vi "rus fit - write RPR line.vi"(9 "folder path":path, 11 "lorentzian":T1={"Amplitude"=0.0035518868945241954, "omega(0)"=2372.1004391165757, "Gamma"=0.8336723020896565, "phase"=3.2843535262399524, "Q"=2845.3631398941097, "Norm  Ampl"=0.37874134839899876, "z (inf)"=0.04739549353095661-0.43244178436899827i, "4corners"={"z (-pi/2)"=-0.4669245429896878-0.04739549353095661i, "z(inf)"=0.04739549353095661-0.43244178436899827i, "z (pi/2)"=0.43244178436899827+0.08187825215164611i, "z center"=-0.01724137931034475+0.01724137931034475i, "z(0)"=-0.08187825215164611+0.4669245429896878i, "radius"=0.45430482390941584}} {"z (inf)" format="%#9_9f"; "Q" format="%#9_9f"; "phase" format="%#9_9f"; "Gamma" format="%#9_9f"; "omega(0)" format="%#9_9f"}) -> ()   [LabVIEW 2015]
uses:
  lorentzian.ctl
  circle corners.ctl
  <vilib>/Utility/file.llb/Write To Spreadsheet File (string).vi
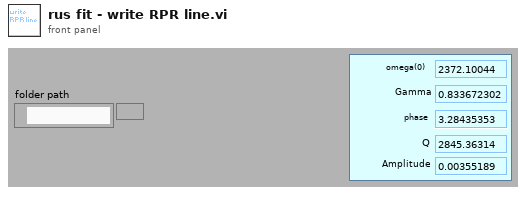
[diagram p1: front panel]
types:
  T1 = typedef "lorentzian.ctl" = cluster{"Amplitude":dbl, "omega(0)":dbl, "Gamma":dbl, "phase":dbl, "Q":dbl, "Norm  Ampl":dbl, "z (inf)":cdb, "4corners":T2}
  T2 = typedef "circle corners.ctl" = cluster{"z (-pi/2)":cdb, "z(inf)":cdb, "z (pi/2)":cdb, "z center":cdb, "z(0)":cdb, "radius":dbl}
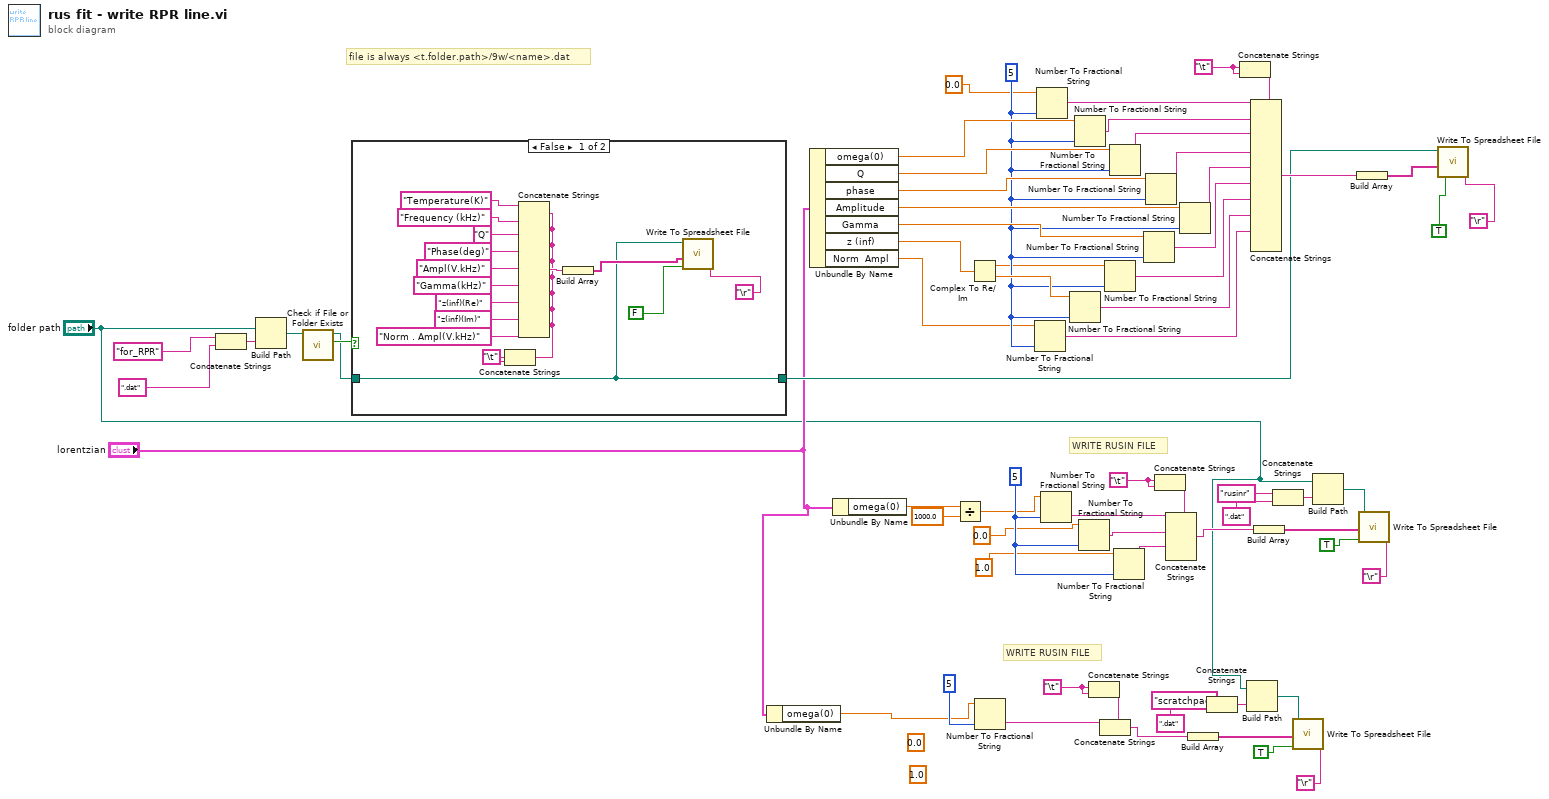
[diagram p0: block diagram]
diagram:
  (unwired) 1.0
  (unwired) 0.0
  w13 = "\t"
  w31 = "\t"
  w29 = i16 5 ("precision (6)")
  w55 = "\t"
  w47 = i16 5 ("precision (6)")
  # "WRITE RUSIN FILE"
  # "WRITE RUSIN FILE"
  # "file is always <t.folder.path>/9w/<name>.dat"
  n1 = Concatenate Strings("for_RPR", ".dat") -> (w63:string)
  n2 = Build Path(base path="folder path", name or relative path=w63) -> (appended path=w39:path)
  n3 = call <vilib>:"Check if File or Folder Exists.vi"("path"=w39) -> ("file or folder exists?"=w38:bool, "dup path"=w37:path)  [unwired: 8 in, 1 out]
  n4 = case shown="False" w38 {
    tunnel: w37 -> [w68 w84]
    tunnel: [w68 w84] -> w36
    frame False {
      w77 = "\t"
      n5 = Concatenate Strings(w77, w77) -> (w72:string)
      n6 = Concatenate Strings("Temperature(K)", w72, "Frequency (kHz)", w72, "Q", w72, "Phase(deg)", w72, "Ampl(V.kHz)", w72, "Gamma(kHz)", w72, "z(inf)(Re)", w72, "z(inf)(Im)", w72, "Norm . Ampl(V.kHz)") -> (w78:string)
      n7 = Build Array(w78) -> (w69:string[])
      n8 = call-poly <vilib>:"Write To Spreadsheet File.vi"("delimiter (\\t)"="\r", "append to file? (new file:F)"=FALSE, "1D data"=w69, "file path (dialog if empty)"=w68) -> ()  [unwired: 4 in, 1 out]
    }
    frame True {
    }
  }
  n9 = Unbundle By Name("lorentzian") -> ("omega(0)"=w1:dbl)
  n10 = Unbundle By Name("lorentzian") -> ("omega(0)"=w61:dbl, "Q"=w58:dbl, "phase"=w57:dbl, "Amplitude"=w56:dbl, "Gamma"=w49:dbl, "z (inf)"=w44:cdb, "Norm  Ampl"=w43:dbl)
  n11 = Unbundle By Name("lorentzian") -> ("omega(0)"=w18:dbl)
  n12 = Divide(x=w18, y=1000.0) -> (x/y=w16:dbl)
  n13 = Complex To Re/Im(x + iy=w44) -> (x=w42:dbl, y=w48:dbl)
  n14 = Number To Fractional String(number=w1, precision (6)=i16 5) -> (F-format string=w15:string)  [unwired: 2 in]
  n15 = Number To Fractional String(number=w43, precision (6)=w47) -> (F-format string=w45:string)  [unwired: 2 in]
  n16 = Number To Fractional String(number=0.0, precision (6)=w47) -> (F-format string=w62:string)  [unwired: 2 in]
  n17 = Number To Fractional String(number=w16, precision (6)=w29) -> (F-format string=w34:string)  [unwired: 2 in]
  n18 = Number To Fractional String(number=w48, precision (6)=w47) -> (F-format string=w46:string)  [unwired: 2 in]
  n19 = Number To Fractional String(number=w61, precision (6)=w47) -> (F-format string=w60:string)  [unwired: 2 in]
  n20 = Number To Fractional String(number=0.0, precision (6)=w29) -> (F-format string=w33:string)  [unwired: 2 in]
  n21 = Concatenate Strings(w13, w13) -> (w11:string)
  n22 = Concatenate Strings(w15, w11) -> (w14:string)
  n23 = Number To Fractional String(number=w42, precision (6)=w47) -> (F-format string=w50:string)  [unwired: 2 in]
  n24 = Number To Fractional String(number=w58, precision (6)=w47) -> (F-format string=w52:string)  [unwired: 2 in]
  n25 = Number To Fractional String(number=1.0, precision (6)=w29) -> (F-format string=w30:string)  [unwired: 2 in]
  n26 = Number To Fractional String(number=w49, precision (6)=w47) -> (F-format string=w51:string)  [unwired: 2 in]
  n27 = Number To Fractional String(number=w57, precision (6)=w47) -> (F-format string=w53:string)  [unwired: 2 in]
  n28 = Concatenate Strings(w31, w31) -> (w28:string)
  n29 = Concatenate Strings(w34, w28, w33, w28, w30, w28) -> (w32:string)
  n30 = Number To Fractional String(number=w56, precision (6)=w47) -> (F-format string=w54:string)  [unwired: 2 in]
  n31 = Build Array(w14) -> (w4:string[])
  n32 = Concatenate Strings("scratchpad", ".dat") -> (w8:string)
  n33 = Concatenate Strings(w55, w55) -> (w41:string)
  n34 = Build Path(base path="folder path", name or relative path=w8) -> (appended path=w5:path)
  n35 = Concatenate Strings(w62, w41, w60, w41, w52, w41, w53, w41, w54, w41, w51, w41, w50, w41, w46, w41, w45, w41, w41) -> (w59:string)
  n36 = Build Array(w32) -> (w21:string[])
  n37 = Concatenate Strings("rusinr", ".dat") -> (w25:string)
  n38 = call-poly <vilib>:"Write To Spreadsheet File.vi"("delimiter (\\t)"="\r", "append to file? (new file:F)"=TRUE, "1D data"=w4, "file path (dialog if empty)"=w5) -> ()  [unwired: 4 in, 1 out]
  n39 = Build Path(base path="folder path", name or relative path=w25) -> (appended path=w22:path)
  n40 = Build Array(w59) -> (w35:string[])
  n41 = call-poly <vilib>:"Write To Spreadsheet File.vi"("delimiter (\\t)"="\r", "append to file? (new file:F)"=TRUE, "1D data"=w21, "file path (dialog if empty)"=w22) -> ()  [unwired: 4 in, 1 out]
  n42 = call-poly <vilib>:"Write To Spreadsheet File.vi"("delimiter (\\t)"="\r", "append to file? (new file:F)"=TRUE, "1D data"=w35, "file path (dialog if empty)"=w36) -> ()  [unwired: 4 in, 1 out]
